vi "Compare endian values subVI.vi"(8 "error in (no error)":errorcluster, 10 "Numeric":dbl format="%#_13g", 11 "Endian":T1) -> (0 "error out":errorcluster, 3 "Values Out":u8[][](array[numeric]))   [LabVIEW 2018, in "Instrument Addon Unit Tests.lvclass"]
uses:
  Instrument Addon Unit Tests.lvclass
  Addon/Addon Shared/Types/Endian.ctl
  Addon/Addon Shared/Types/Type Cast Type.ctl
  Addon/Addon Shared/Types/Metadata Channel Type.ctl
  Addon/Addon Engine/Instrument Addon Engine.lvlib
  Addon/Addon Shared/Instrument Addon Shared.lvlib
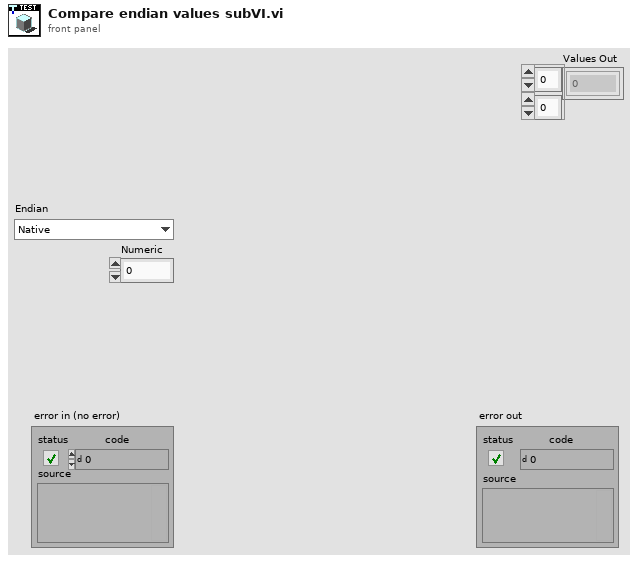
[diagram p1: front panel]
types:
  T1 = typedef "Instrument Addon Shared.lvlib/Endian.ctl" = enum16{"Native", "Little", "Big"}
  T2 = typedef "Instrument Addon Shared.lvlib/Type Cast Type.ctl" = enum16{"DBL", "SGL", "U64", "U32", "U16", "U8", "I64", "I32", "I16", "I8"}
  T3 = typedef "Instrument Addon Shared.lvlib/Metadata Channel Type.ctl" = enum16{"Enumerated List", "Format", "Type Cast"}
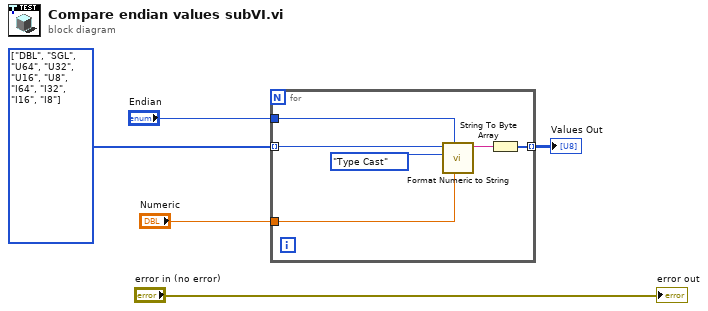
[diagram p0: block diagram]
diagram:
  w5 = T2[] [enum."DBL", enum."SGL", enum."U64", enum."U32", enum."U16", enum."U8", enum."I64", enum."I32", enum."I16", enum."I8"] items=["DBL", "SGL", "U64", "U32", "U16", "U8", "I64", "I32", "I16", "I8"]
  n1 = for {
    tunnel: w5 -> [w9] mode=indexing
    tunnel: "Endian" -> [w11]
    tunnel: "Numeric" -> [w7]
    tunnel: [w6] -> w1 mode=indexing
    n2 = call "Format Numeric to String.vi"("Numeric"=w7, "Endian"=w11, "Channel Type"=Metadata_Channel_Type."Type Cast", "Type"=w9) -> ("Value"=w8:string)  [unwired: 7 in]
    n3 = String To Byte Array(string=w8) -> (unsigned byte array=w6:u8[])
  }
  "Values Out" <- w1
  "error out" <- "error in (no error)"
